vi "Victor8246_Link.vi"(4 "错误输入":errorcluster caption="错误输入（无错误）", 7 "MyIndex":u8) -> (0 "错误输出":errorcluster, 3 "OK?":bool)   [LabVIEW 2015, in "Victor8246.lvlib"]
uses:
  Victor8246.lvlib
  <vilib>/Instr/_visa.llb/VISA Configure Serial Port (Instr).vi
panel:
  out "VISA资源名称输出":refnum<visa-resource-name>
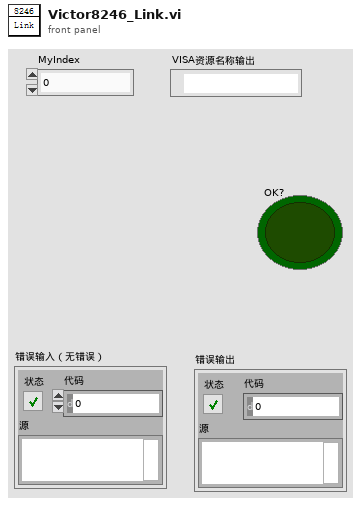
[diagram p1: front panel]
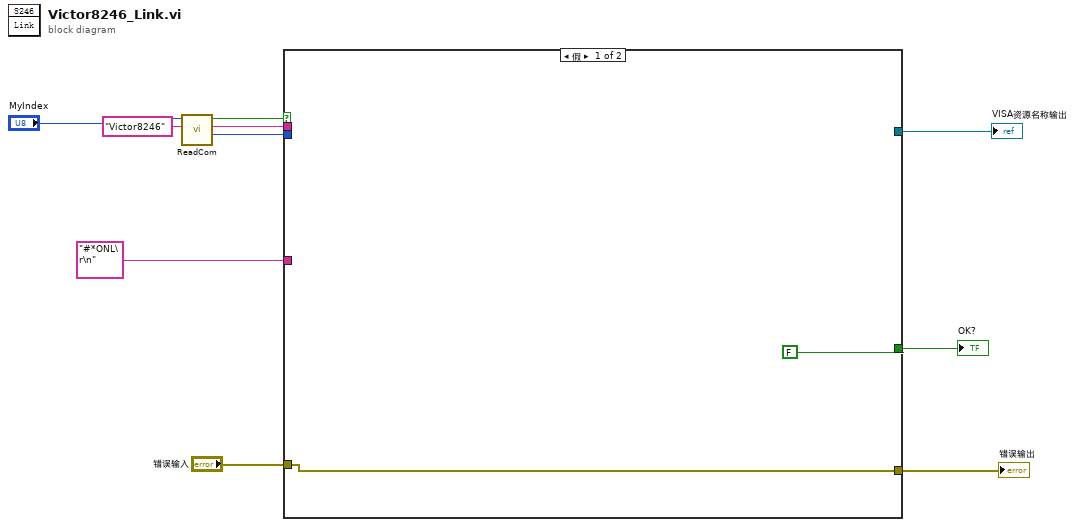
[diagram p0: block diagram]
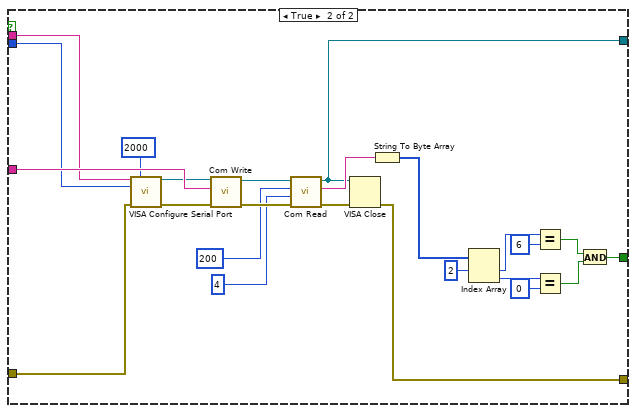
[diagram p2: hidden frame]
diagram:
  n1 = call "ReadCom.vi"("仪器名称"="Victor8246", "MyIndex"="MyIndex") -> ("Baudrate"=w5:i32, "COM"=w6:string, "OK?"=w4:bool)  [unwired: 7 in]
  n2 = case shown="假" w4 {
    tunnel: [FALSE w29] -> w10
    tunnel: "错误输入" -> [w11 w27]
    tunnel: "#*ONL\r\n" ("字符串") -> [_ w26]
    tunnel: w6 -> [_ w18]
    tunnel: w5 -> [_ w17]
    tunnel: [w11 w14] -> w3
    tunnel: [_ w13] -> w2
    frame False {
    }
    frame True {
      n3 = call-poly "VISA Configure Serial Port"("VISA resource name"=w18, "timeout (10sec)"=u32 2000, "baud rate (9600)"=w17, "error in (no error)"=w27) -> ("VISA resource name out"=w15:refnum<visa-resource-name>, "error out"=w19:errorcluster)  [unwired: 10 in]
      n4 = call "Com Write.vi"("错误输入（无错误）"=w19, "Wbuff"=w26, "VISA In"=w15) -> ("错误输出"=w25:errorcluster, "VISA Out"=w24:refnum<visa-resource-name>)  [unwired: 7 in]
      n5 = call "Com Read.vi"("错误输入（无错误）"=w25, "num"=u32 4, "超时"=u32 200, "VISA In"=w24) -> ("错误输出"=w20:errorcluster, "buff"=w21:string, "VISA Out"=w13:refnum<visa-resource-name>)  [unwired: 5 in]
      n6 = VISA Close(VISA resource name=w13, error in (no error)=w20) -> (error out=w14:errorcluster)
      n7 = String To Byte Array(string=w21) -> (unsigned byte array=w28:u8[])
      n8 = Index Array(array=w28, index #1=2 ("索引")) -> (element #1=w35:u8, element #2=w32:u8)  [unwired: 1 in]
      n9 = Equal?(x=w35, y=u8 6) -> (x = y?=w31:bool)
      n10 = Equal?(x=w32, y=u8 0) -> (x = y?=w30:bool)
      n11 = And(x=w31, y=w30) -> (x .and. y?=w29:bool)
    }
  }
  "OK?" <- w10
  "错误输出" <- w3
  "VISA资源名称输出" <- w2
